vi "RW PI Parameters.vi"(0 "Path":path, 2 "Read (F)":bool, 7 "PI Parameters In":T1, 11 "Error In":errorcluster) -> (8 "PI Parameters Out":T1, 15 "Error Out":errorcluster)   [LabVIEW 2013]
uses:
  TypeDef/PI Parameters.ctl
  <vilib>/Utility/config.llb/Read Key (Double).vi
  <vilib>/Utility/config.llb/Write Key (Double).vi
  <vilib>/Utility/config.llb/NI_LVConfig.lvlib
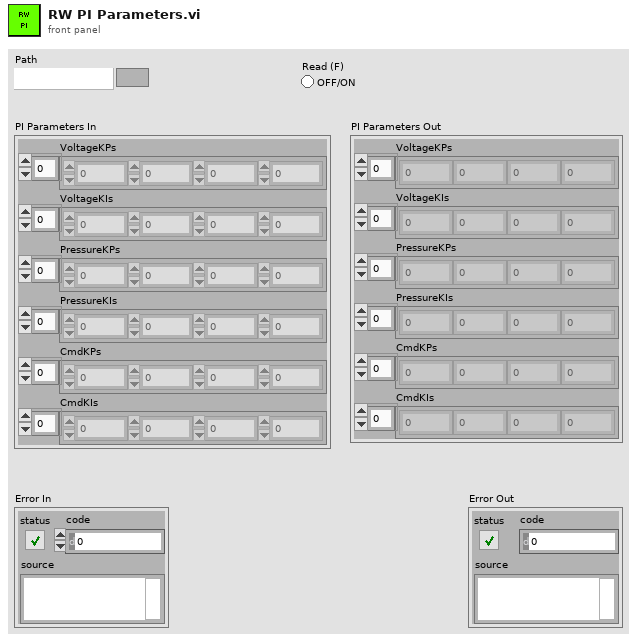
[diagram p1: front panel]
types:
  T1 = typedef "PI Parameters.ctl" = cluster{"VoltageKPs":dbl[], "VoltageKIs":dbl[], "PressureKPs":dbl[], "PressureKIs":dbl[], "CmdKPs":dbl[], "CmdKIs":dbl[]}
  T2 = typedef "NI_LVConfig.lvlib/Config Data RefNum.ctl" = refnum<k1>
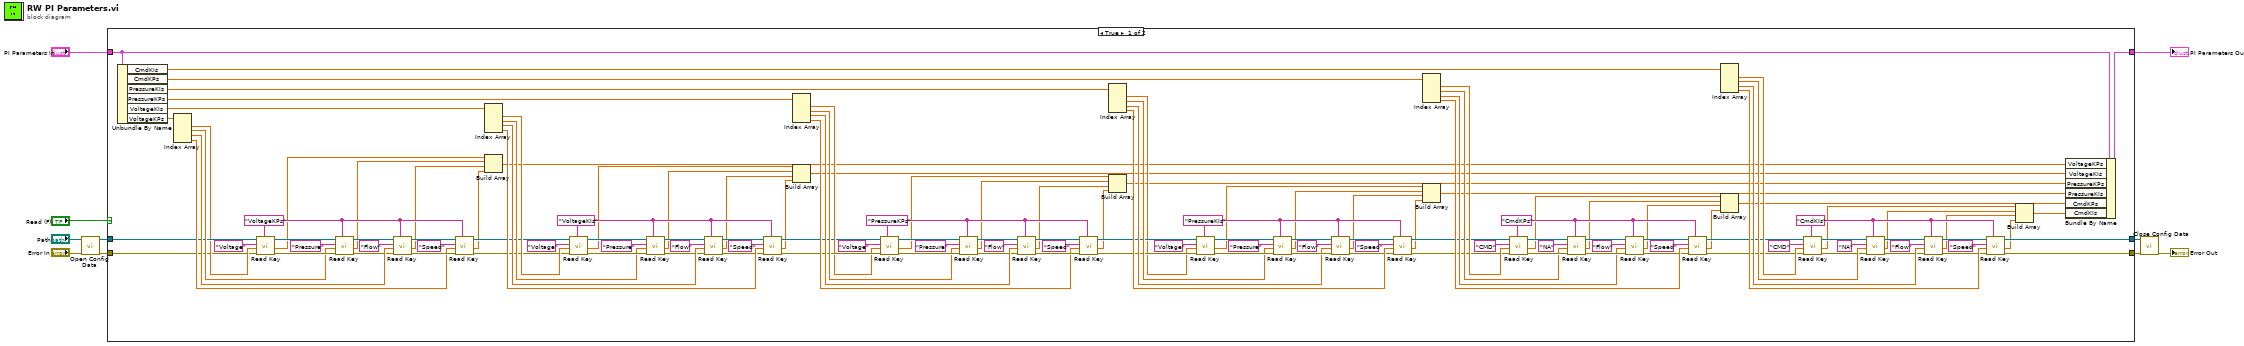
[diagram p0: block diagram]
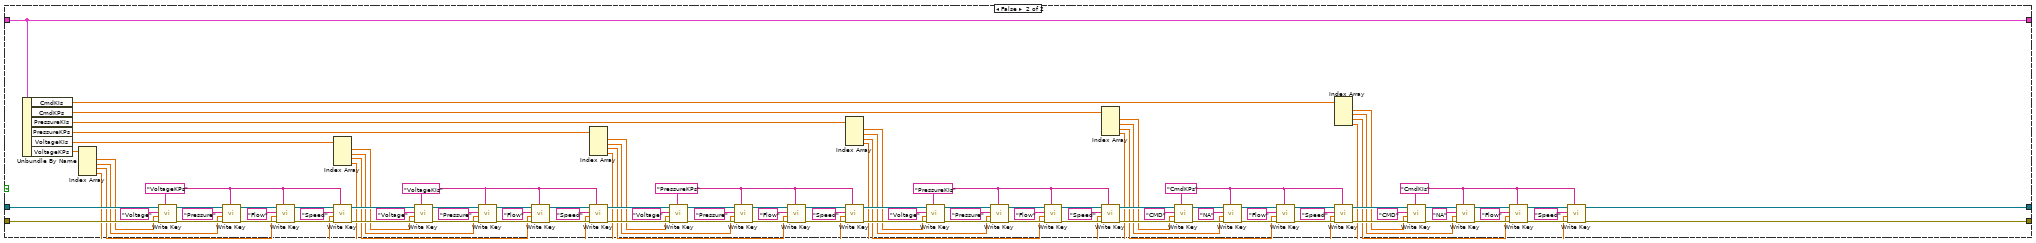
[diagram p2: hidden frame]
diagram:
  n1 = call <vilib>:"Open Config Data.vi"("error in (no error)"="Error In", "configuration file path"="Path") -> ("error out"=w6:errorcluster, "refnum"=w7:T2)  [unwired: 7 in, 1 out]
  n2 = case shown="True" "Read (F)" {
    tunnel: w7 -> [w68 w263]
    tunnel: w6 -> [w65 w262]
    tunnel: "PI Parameters In" -> [w15 w201]
    tunnel: [w139 w208] -> w4
    tunnel: [w142 w247] -> w3
    tunnel: [w14 w201] -> w1
    frame True {
      w63 = "CmdKIs"
      w143 = "CmdKPs"
      w144 = "PressureKIs"
      w145 = "PressureKPs"
      w146 = "VoltageKIs"
      w147 = "VoltageKPs"
      n3 = Unbundle By Name(w15) -> ("CmdKIs"=w40:dbl[], "CmdKPs"=w148:dbl[], "PressureKIs"=w149:dbl[], "PressureKPs"=w150:dbl[], "VoltageKIs"=w151:dbl[], "VoltageKPs"=w152:dbl[])
      n4 = Index Array(array=w152) -> (element #1=w66:dbl, element #2=w70:dbl, element #3=w73:dbl, element #4=w76:dbl)  [unwired: 4 in]
      n5 = call-poly <vilib>:"Read Key.vi"("section"=w147, "error in (no error)"=w65, "default value"=w66, "key"="Voltage", "refnum"=w68) -> ("error out"=w71:errorcluster, "value"=w38:dbl, "refnum out"=w64:T2)  [unwired: 3 in, 1 out]
      n6 = call-poly <vilib>:"Read Key.vi"("section"=w147, "error in (no error)"=w71, "default value"=w70, "key"="Pressure", "refnum"=w64) -> ("error out"=w72:errorcluster, "value"=w37:dbl, "refnum out"=w62:T2)  [unwired: 3 in, 1 out]
      n7 = call-poly <vilib>:"Read Key.vi"("section"=w147, "error in (no error)"=w72, "default value"=w73, "key"="Flow", "refnum"=w62) -> ("error out"=w77:errorcluster, "value"=w36:dbl, "refnum out"=w61:T2)  [unwired: 3 in, 1 out]
      n8 = call-poly <vilib>:"Read Key.vi"("section"=w147, "error in (no error)"=w77, "default value"=w76, "key"="Speed", "refnum"=w61) -> ("error out"=w78:errorcluster, "value"=w35:dbl, "refnum out"=w60:T2)  [unwired: 3 in, 1 out]
      n9 = Index Array(array=w151) -> (element #1=w79:dbl, element #2=w82:dbl, element #3=w85:dbl, element #4=w88:dbl)  [unwired: 4 in]
      n10 = Build Array(w38, w37, w36, w35) -> (w11:dbl[])
      n11 = call-poly <vilib>:"Read Key.vi"("section"=w146, "error in (no error)"=w78, "default value"=w79, "key"="Voltage", "refnum"=w60) -> ("error out"=w83:errorcluster, "value"=w34:dbl, "refnum out"=w59:T2)  [unwired: 3 in, 1 out]
      n12 = call-poly <vilib>:"Read Key.vi"("section"=w146, "error in (no error)"=w83, "default value"=w82, "key"="Pressure", "refnum"=w59) -> ("error out"=w84:errorcluster, "value"=w33:dbl, "refnum out"=w58:T2)  [unwired: 3 in, 1 out]
      n13 = call-poly <vilib>:"Read Key.vi"("section"=w146, "error in (no error)"=w84, "default value"=w85, "key"="Flow", "refnum"=w58) -> ("error out"=w87:errorcluster, "value"=w32:dbl, "refnum out"=w57:T2)  [unwired: 3 in, 1 out]
      n14 = call-poly <vilib>:"Read Key.vi"("section"=w146, "error in (no error)"=w87, "default value"=w88, "key"="Speed", "refnum"=w57) -> ("error out"=w92:errorcluster, "value"=w31:dbl, "refnum out"=w56:T2)  [unwired: 3 in, 1 out]
      n15 = Index Array(array=w150) -> (element #1=w91:dbl, element #2=w94:dbl, element #3=w97:dbl, element #4=w100:dbl)  [unwired: 4 in]
      n16 = Build Array(w34, w33, w32, w31) -> (w12:dbl[])
      n17 = call-poly <vilib>:"Read Key.vi"("section"=w145, "error in (no error)"=w92, "default value"=w91, "key"="Voltage", "refnum"=w56) -> ("error out"=w95:errorcluster, "value"=w30:dbl, "refnum out"=w55:T2)  [unwired: 3 in, 1 out]
      n18 = call-poly <vilib>:"Read Key.vi"("section"=w145, "error in (no error)"=w95, "default value"=w94, "key"="Pressure", "refnum"=w55) -> ("error out"=w96:errorcluster, "value"=w29:dbl, "refnum out"=w54:T2)  [unwired: 3 in, 1 out]
      n19 = call-poly <vilib>:"Read Key.vi"("section"=w145, "error in (no error)"=w96, "default value"=w97, "key"="Flow", "refnum"=w54) -> ("error out"=w101:errorcluster, "value"=w28:dbl, "refnum out"=w53:T2)  [unwired: 3 in, 1 out]
      n20 = call-poly <vilib>:"Read Key.vi"("section"=w145, "error in (no error)"=w101, "default value"=w100, "key"="Speed", "refnum"=w53) -> ("error out"=w103:errorcluster, "value"=w27:dbl, "refnum out"=w52:T2)  [unwired: 3 in, 1 out]
      n21 = Index Array(array=w149) -> (element #1=w39:dbl, element #2=w105:dbl, element #3=w108:dbl, element #4=w111:dbl)  [unwired: 4 in]
      n22 = Build Array(w30, w29, w28, w27) -> (w13:dbl[])
      n23 = call-poly <vilib>:"Read Key.vi"("section"=w144, "error in (no error)"=w103, "default value"=w39, "key"="Voltage", "refnum"=w52) -> ("error out"=w106:errorcluster, "value"=w26:dbl, "refnum out"=w51:T2)  [unwired: 3 in, 1 out]
      n24 = call-poly <vilib>:"Read Key.vi"("section"=w144, "error in (no error)"=w106, "default value"=w105, "key"="Pressure", "refnum"=w51) -> ("error out"=w109:errorcluster, "value"=w25:dbl, "refnum out"=w50:T2)  [unwired: 3 in, 1 out]
      n25 = call-poly <vilib>:"Read Key.vi"("section"=w144, "error in (no error)"=w109, "default value"=w108, "key"="Flow", "refnum"=w50) -> ("error out"=w110:errorcluster, "value"=w24:dbl, "refnum out"=w49:T2)  [unwired: 3 in, 1 out]
      n26 = call-poly <vilib>:"Read Key.vi"("section"=w144, "error in (no error)"=w110, "default value"=w111, "key"="Speed", "refnum"=w49) -> ("error out"=w113:errorcluster, "value"=w23:dbl, "refnum out"=w48:T2)  [unwired: 3 in, 1 out]
      n27 = Index Array(array=w148) -> (element #1=w114:dbl, element #2=w117:dbl, element #3=w120:dbl, element #4=w124:dbl)  [unwired: 4 in]
      n28 = Build Array(w26, w25, w24, w23) -> (w16:dbl[])
      n29 = call-poly <vilib>:"Read Key.vi"("section"=w143, "error in (no error)"=w113, "default value"=w114, "key"="CMD", "refnum"=w48) -> ("error out"=w118:errorcluster, "value"=w19:dbl, "refnum out"=w47:T2)  [unwired: 3 in, 1 out]
      n30 = call-poly <vilib>:"Read Key.vi"("section"=w143, "error in (no error)"=w118, "default value"=w117, "key"="NA", "refnum"=w47) -> ("error out"=w121:errorcluster, "value"=w20:dbl, "refnum out"=w46:T2)  [unwired: 3 in, 1 out]
      n31 = call-poly <vilib>:"Read Key.vi"("section"=w143, "error in (no error)"=w121, "default value"=w120, "key"="Flow", "refnum"=w46) -> ("error out"=w122:errorcluster, "value"=w21:dbl, "refnum out"=w45:T2)  [unwired: 3 in, 1 out]
      n32 = call-poly <vilib>:"Read Key.vi"("section"=w143, "error in (no error)"=w122, "default value"=w124, "key"="Speed", "refnum"=w45) -> ("error out"=w126:errorcluster, "value"=w22:dbl, "refnum out"=w125:T2)  [unwired: 3 in, 1 out]
      n33 = Index Array(array=w40) -> (element #1=w127:dbl, element #2=w131:dbl, element #3=w135:dbl, element #4=w141:dbl)  [unwired: 4 in]
      n34 = Build Array(w19, w20, w21, w22) -> (w17:dbl[])
      n35 = call-poly <vilib>:"Read Key.vi"("section"=w63, "error in (no error)"=w126, "default value"=w127, "key"="CMD", "refnum"=w125) -> ("error out"=w130:errorcluster, "value"=w44:dbl, "refnum out"=w129:T2)  [unwired: 3 in, 1 out]
      n36 = call-poly <vilib>:"Read Key.vi"("section"=w63, "error in (no error)"=w130, "default value"=w131, "key"="NA", "refnum"=w129) -> ("error out"=w134:errorcluster, "value"=w43:dbl, "refnum out"=w133:T2)  [unwired: 3 in, 1 out]
      n37 = call-poly <vilib>:"Read Key.vi"("section"=w63, "error in (no error)"=w134, "default value"=w135, "key"="Flow", "refnum"=w133) -> ("error out"=w137:errorcluster, "value"=w42:dbl, "refnum out"=w138:T2)  [unwired: 3 in, 1 out]
      n38 = call-poly <vilib>:"Read Key.vi"("section"=w63, "error in (no error)"=w137, "default value"=w141, "key"="Speed", "refnum"=w138) -> ("error out"=w142:errorcluster, "value"=w41:dbl, "refnum out"=w139:T2)  [unwired: 3 in, 1 out]
      n39 = Build Array(w44, w43, w42, w41) -> (w18:dbl[])
      n40 = Bundle By Name(cluster=w15, "VoltageKPs"=w11, "VoltageKIs"=w12, "PressureKPs"=w13, "PressureKIs"=w16, "CmdKPs"=w17, "CmdKIs"=w18) -> (w14:T1)
    }
    frame False {
      w261 = "CmdKIs"
      w260 = "CmdKPs"
      w259 = "PressureKIs"
      w258 = "PressureKPs"
      w257 = "VoltageKIs"
      w256 = "VoltageKPs"
      n41 = Unbundle By Name(w201) -> ("CmdKIs"=w207:dbl[], "CmdKPs"=w202:dbl[], "PressureKIs"=w203:dbl[], "PressureKPs"=w204:dbl[], "VoltageKIs"=w205:dbl[], "VoltageKPs"=w206:dbl[])
      n42 = Index Array(array=w206) -> (element #1=w197:dbl, element #2=w198:dbl, element #3=w199:dbl, element #4=w200:dbl)  [unwired: 4 in]
      n43 = call-poly <vilib>:"Write Key.vi"("section"=w256, "error in (no error)"=w262, "value"=w197, "key"="Voltage", "refnum"=w263) -> ("error out"=w246:errorcluster, "refnum out"=w245:T2)  [unwired: 4 in, 1 out]
      n44 = call-poly <vilib>:"Write Key.vi"("section"=w256, "error in (no error)"=w246, "value"=w198, "key"="Pressure", "refnum"=w245) -> ("error out"=w243:errorcluster, "refnum out"=w244:T2)  [unwired: 4 in, 1 out]
      n45 = call-poly <vilib>:"Write Key.vi"("section"=w256, "error in (no error)"=w243, "value"=w199, "key"="Flow", "refnum"=w244) -> ("error out"=w242:errorcluster, "refnum out"=w241:T2)  [unwired: 4 in, 1 out]
      n46 = Index Array(array=w205) -> (element #1=w169:dbl, element #2=w170:dbl, element #3=w171:dbl, element #4=w172:dbl)  [unwired: 4 in]
      n47 = call-poly <vilib>:"Write Key.vi"("section"=w256, "error in (no error)"=w242, "value"=w200, "key"="Speed", "refnum"=w241) -> ("error out"=w239:errorcluster, "refnum out"=w240:T2)  [unwired: 4 in, 1 out]
      n48 = call-poly <vilib>:"Write Key.vi"("section"=w257, "error in (no error)"=w239, "value"=w169, "key"="Voltage", "refnum"=w240) -> ("error out"=w237:errorcluster, "refnum out"=w238:T2)  [unwired: 4 in, 1 out]
      n49 = call-poly <vilib>:"Write Key.vi"("section"=w257, "error in (no error)"=w237, "value"=w170, "key"="Pressure", "refnum"=w238) -> ("error out"=w235:errorcluster, "refnum out"=w236:T2)  [unwired: 4 in, 1 out]
      n50 = call-poly <vilib>:"Write Key.vi"("section"=w257, "error in (no error)"=w235, "value"=w171, "key"="Flow", "refnum"=w236) -> ("error out"=w234:errorcluster, "refnum out"=w233:T2)  [unwired: 4 in, 1 out]
      n51 = Index Array(array=w204) -> (element #1=w165:dbl, element #2=w166:dbl, element #3=w167:dbl, element #4=w168:dbl)  [unwired: 4 in]
      n52 = call-poly <vilib>:"Write Key.vi"("section"=w257, "error in (no error)"=w234, "value"=w172, "key"="Speed", "refnum"=w233) -> ("error out"=w231:errorcluster, "refnum out"=w232:T2)  [unwired: 4 in, 1 out]
      n53 = call-poly <vilib>:"Write Key.vi"("section"=w258, "error in (no error)"=w231, "value"=w165, "key"="Voltage", "refnum"=w232) -> ("error out"=w229:errorcluster, "refnum out"=w230:T2)  [unwired: 4 in, 1 out]
      n54 = call-poly <vilib>:"Write Key.vi"("section"=w258, "error in (no error)"=w229, "value"=w166, "key"="Pressure", "refnum"=w230) -> ("error out"=w228:errorcluster, "refnum out"=w227:T2)  [unwired: 4 in, 1 out]
      n55 = call-poly <vilib>:"Write Key.vi"("section"=w258, "error in (no error)"=w228, "value"=w167, "key"="Flow", "refnum"=w227) -> ("error out"=w226:errorcluster, "refnum out"=w225:T2)  [unwired: 4 in, 1 out]
      n56 = Index Array(array=w203) -> (element #1=w162:dbl, element #2=w161:dbl, element #3=w163:dbl, element #4=w164:dbl)  [unwired: 4 in]
      n57 = call-poly <vilib>:"Write Key.vi"("section"=w258, "error in (no error)"=w226, "value"=w168, "key"="Speed", "refnum"=w225) -> ("error out"=w223:errorcluster, "refnum out"=w224:T2)  [unwired: 4 in, 1 out]
      n58 = call-poly <vilib>:"Write Key.vi"("section"=w259, "error in (no error)"=w223, "value"=w162, "key"="Voltage", "refnum"=w224) -> ("error out"=w221:errorcluster, "refnum out"=w222:T2)  [unwired: 4 in, 1 out]
      n59 = call-poly <vilib>:"Write Key.vi"("section"=w259, "error in (no error)"=w221, "value"=w161, "key"="Pressure", "refnum"=w222) -> ("error out"=w219:errorcluster, "refnum out"=w220:T2)  [unwired: 4 in, 1 out]
      n60 = call-poly <vilib>:"Write Key.vi"("section"=w259, "error in (no error)"=w219, "value"=w163, "key"="Flow", "refnum"=w220) -> ("error out"=w218:errorcluster, "refnum out"=w217:T2)  [unwired: 4 in, 1 out]
      n61 = Index Array(array=w202) -> (element #1=w157:dbl, element #2=w158:dbl, element #3=w159:dbl, element #4=w160:dbl)  [unwired: 4 in]
      n62 = call-poly <vilib>:"Write Key.vi"("section"=w259, "error in (no error)"=w218, "value"=w164, "key"="Speed", "refnum"=w217) -> ("error out"=w255:errorcluster, "refnum out"=w216:T2)  [unwired: 4 in, 1 out]
      n63 = call-poly <vilib>:"Write Key.vi"("section"=w260, "error in (no error)"=w255, "value"=w157, "key"="CMD", "refnum"=w216) -> ("error out"=w254:errorcluster, "refnum out"=w215:T2)  [unwired: 4 in, 1 out]
      n64 = call-poly <vilib>:"Write Key.vi"("section"=w260, "error in (no error)"=w254, "value"=w158, "key"="NA", "refnum"=w215) -> ("error out"=w253:errorcluster, "refnum out"=w214:T2)  [unwired: 4 in, 1 out]
      n65 = call-poly <vilib>:"Write Key.vi"("section"=w260, "error in (no error)"=w253, "value"=w159, "key"="Flow", "refnum"=w214) -> ("error out"=w252:errorcluster, "refnum out"=w213:T2)  [unwired: 4 in, 1 out]
      n66 = Index Array(array=w207) -> (element #1=w153:dbl, element #2=w154:dbl, element #3=w155:dbl, element #4=w156:dbl)  [unwired: 4 in]
      n67 = call-poly <vilib>:"Write Key.vi"("section"=w260, "error in (no error)"=w252, "value"=w160, "key"="Speed", "refnum"=w213) -> ("error out"=w251:errorcluster, "refnum out"=w212:T2)  [unwired: 4 in, 1 out]
      n68 = call-poly <vilib>:"Write Key.vi"("section"=w261, "error in (no error)"=w251, "value"=w153, "key"="CMD", "refnum"=w212) -> ("error out"=w250:errorcluster, "refnum out"=w211:T2)  [unwired: 4 in, 1 out]
      n69 = call-poly <vilib>:"Write Key.vi"("section"=w261, "error in (no error)"=w250, "value"=w154, "key"="NA", "refnum"=w211) -> ("error out"=w249:errorcluster, "refnum out"=w210:T2)  [unwired: 4 in, 1 out]
      n70 = call-poly <vilib>:"Write Key.vi"("section"=w261, "error in (no error)"=w249, "value"=w155, "key"="Flow", "refnum"=w210) -> ("error out"=w248:errorcluster, "refnum out"=w209:T2)  [unwired: 4 in, 1 out]
      n71 = call-poly <vilib>:"Write Key.vi"("section"=w261, "error in (no error)"=w248, "value"=w156, "key"="Speed", "refnum"=w209) -> ("error out"=w247:errorcluster, "refnum out"=w208:T2)  [unwired: 4 in, 1 out]
    }
  }
  "PI Parameters Out" <- w1
  n72 = call <vilib>:"Close Config Data.vi"("error in (no error)"=w3, "refnum"=w4) -> ("error out"=→"Error Out":errorcluster)  [unwired: 8 in, 1 out]
